vi "Configure Power Analysis (Slew Rate).vi"(8 "error in (no error)":errorcluster, 10 "Slew Rate Source (0: V)":i32(ring) items=["V", "I"], 11 "VISA resource name":refnum<visa-resource-name>) -> (0 "error out":errorcluster, 3 "VISA resource name out":refnum<visa-resource-name>)   [LabVIEW 2017, in "Agilent 2000 3000 X-Series.lvlib"]
doc: "Applies the slew rate analysis.\n\n<B>Note(s):</B>\nUse <B>Read Measurement (Slew Rate Power Analysis).vi</B> to read the result of this power analysis.\nThis VI is not supported by EDUX1052A/G, DSOX1202A/G, DSOX1204A/G models"
uses:
  Agilent 2000 3000 X-Series.lvlib
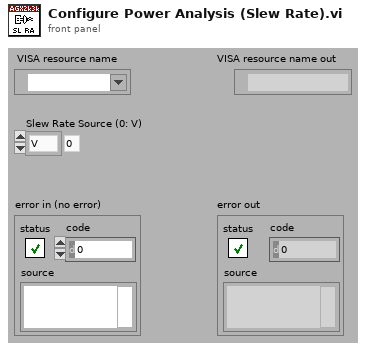
[diagram p1: front panel]
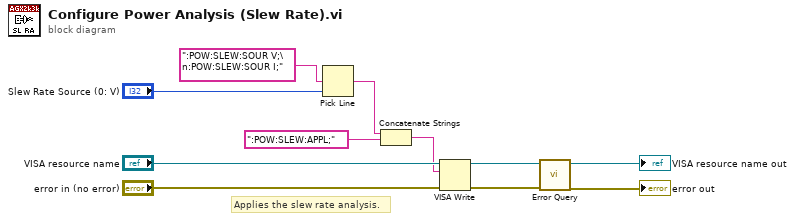
[diagram p0: block diagram]
diagram:
  # "Applies the slew rate analysis."
  n1 = Pick Line(multi-line string=":POW:SLEW:SOUR V;\n:POW:SLEW:SOUR I;", line index="Slew Rate Source (0: V)") -> (output string=w2:string)  [unwired: 1 out]
  n2 = Concatenate Strings(w2, ":POW:SLEW:APPL;") -> (w1:string)
  n3 = VISA Write(VISA resource name="VISA resource name", write buffer=w1, error in (no error)="error in (no error)") -> (VISA resource name out=w7:refnum<visa-resource-name>, error out=w6:errorcluster)  [unwired: 1 out]
  n4 = call "Error Query.vi"("error in (no error)"=w6, "VISA resource name"=w7) -> ("error out"=→"error out":errorcluster, "VISA resource name out"=→"VISA resource name out":refnum<visa-resource-name>)  [unwired: 8 out]
